vi "pump_motor_run.vi"(8 "error in (no error)":errorcluster, 9 "Enable":bool, 10 "Empty Swim Bladder":bool, 11 "PWM Duty Cycle [0, 1]":dbl(slide)=1.0 scale=0.0..1.0) -> (0 "error out":errorcluster, 1 "Driver Error/Pump Motor off":bool, 3 "Motor Current[A]":dbl)   [LabVIEW 2013]
uses:
  My Computer/Controls/Advanced Swimbladder Indicators.ctl
  <vilib>/myRIO/Instrument Drivers/Onboard IO/AI/vis/Smart Open.vi
  <vilib>/myRIO/Instrument Drivers/Onboard IO/AI/vis/Read.vi
  <vilib>/myRIO/Instrument Drivers/Onboard IO/DIO/vis/Smart Open.vi
  <vilib>/myRIO/Instrument Drivers/Onboard IO/DIO/vis/Read.vi
  <vilib>/myRIO/Instrument Drivers/Onboard IO/PWM/vis/Smart Open.vi
  <vilib>/myRIO/Instrument Drivers/Onboard IO/PWM/vis/Set Duty Cycle and Frequency.vi
  <vilib>/myRIO/Instrument Drivers/Onboard IO/DIO/vis/Write.vi
  <vilib>/myRIO/Instrument Drivers/Onboard IO/AI/vis/Open.vi
  <vilib>/myRIO/Instrument Drivers/Onboard IO/DIO/vis/Open.vi
  <vilib>/myRIO/Instrument Drivers/Onboard IO/PWM/vis/Open.vi
  <vilib>/myRIO/Common/Instrument Driver Framework/myRIO v1.0/AI/vis/myRIO v1.1 Open AI.vi
  <vilib>/myRIO/Common/Instrument Driver Framework/myRIO v1.0/DIO/vis/myRIO v1.1 Open DIO.vi
  <vilib>/myRIO/Common/Instrument Driver Framework/myRIO v1.0/PWM/vis/myRIO v1.1 Open PWM.vi
  <vilib>/myRIO/Common/Instrument Driver Framework/Utilities/vis/Validate Channels.vi
  <vilib>/myRIO/Common/Instrument Driver Framework/myRIO v1.0/AI/vis/myRIO v1.0 Reserve AI.vi
  <vilib>/myRIO/Common/Instrument Driver Framework/myRIO v1.0/DIO/vis/myRIO v1.0 Reserve DIO.vi
  <vilib>/myRIO/Common/Instrument Driver Framework/myRIO v1.0/PWM/vis/myRIO v1.0 Reserve PWM.vi
  <vilib>/myRIO/Common/Instrument Driver Framework/myRIO v1.0/AI/vis/myRIO v1.0 Build MUX Configuration AI.vi
  <vilib>/myRIO/Common/Instrument Driver Framework/myRIO v1.0/Resource Manager/vis/myRIO v1.0 Reserve Channel List.vi
  <vilib>/myRIO/Common/Instrument Driver Framework/myRIO v1.0/DIO/vis/myRIO v1.0 Build MUX Configuration DIO.vi
  <vilib>/myRIO/Common/Instrument Driver Framework/myRIO v1.0/PWM/vis/myRIO v1.0 Build MUX Configuration PWM.vi
  <vilib>/myRIO/Common/Instrument Driver Framework/myRIO v1.0/Resource Manager/vis/myRIO v1.0 Reserve Channel.vi
  <vilib>/myRIO/Common/Instrument Driver Framework/myRIO v1.0/Resource Manager/vis/myRIO v1.0 Unreserve Channel.vi
  <vilib>/myRIO/Common/Instrument Driver Framework/myRIO v1.0/Resource Manager/vis/myRIO v1.0 Create Configuration List.vi
  <vilib>/myRIO/Common/Instrument Driver Framework/myRIO v1.0/Resource Manager/vis/myRIO v1.0 Build Mutex Name.vi
  <vilib>/myRIO/Common/Instrument Driver Framework/myRIO v1.0/myRIO v1.1 Open.vi
  <vilib>/myRIO/Common/Instrument Driver Framework/myRIO v1.0/AI/vis/myRIO v1.0 Get Scaling Constants AI.vi
  <vilib>/Utility/VariantDataType/GetNumericInfo.vi
  <vilib>/Utility/error.llb/Error Cluster From Error Code.vi
  <vilib>/myRIO/Common/Instrument Driver Framework/Utilities/vis/IO Manager.vi
  <vilib>/myRIO/Common/Instrument Driver Framework/Utilities/vis/Configuration Manager.vi
  <vilib>/myRIO/Common/Instrument Driver Framework/myRIO v1.0/myRIO v1.0 Close.vi
  <vilib>/myRIO/Common/Instrument Driver Framework/myRIO v1.0/AI/vis/myRIO v1.0 Read AI.vi
  <vilib>/myRIO/Common/Instrument Driver Framework/myRIO v1.0/Resource Manager/vis/myRIO v1.0 Configure IO.vi
  <vilib>/myRIO/Common/Instrument Driver Framework/myRIO v1.0/DIO/vis/myRIO v1.0 Read DIO.vi
  <vilib>/myRIO/Common/Instrument Driver Framework/myRIO v1.0/PWM/vis/myRIO v1.0 Write PWM.vi
  <vilib>/myRIO/Common/Instrument Driver Framework/myRIO v1.0/DIO/vis/myRIO v1.0 Write DIO.vi
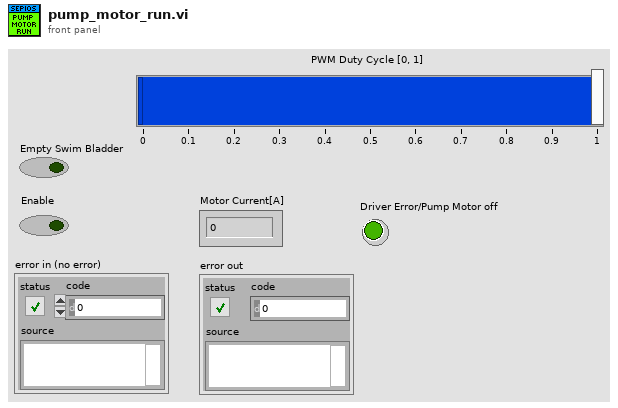
[diagram p1: front panel]
types:
  T1 = typedef "Advanced Swimbladder Indicators.ctl" = cluster{"P_ref [Pa]":dbl, "X_Actual [m]":dbl, "Motor Current[A]":dbl}
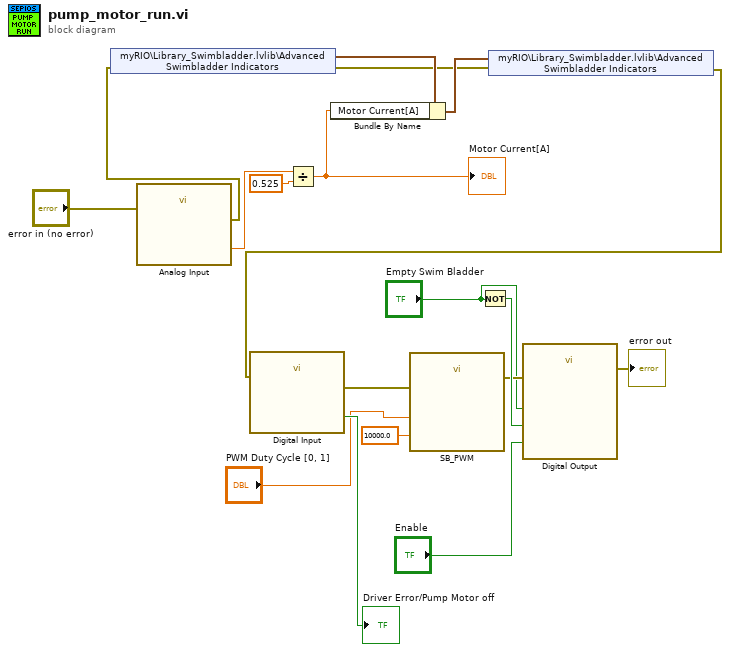
[diagram p0: block diagram]
diagram:
  n1 = call "Analog Input"("error in (no error)"="error in (no error)") -> ("SB_FB (B/AI0 (Pin 3))"=w14:dbl, "error out"=w3:errorcluster)  [unwired: 25 in]
  n2 = shared-variable "myRIO\\Library_Swimbladder.lvlib\\Advanced Swimbladder Indicators"(error in=w3) -> (w6:T1, error out=w2:errorcluster)
  n3 = Divide(x=w14, y=0.525) -> (x/y=w5:dbl)
  "Motor Current[A]" <- w5
  n4 = Bundle By Name(cluster=w6, "Motor Current[A]"=w5) -> (w4:T1)
  n5 = Not(x="Empty Swim Bladder") -> (.not. x?=w18:bool)
  n6 = shared-variable "myRIO\\Library_Swimbladder.lvlib\\Advanced Swimbladder Indicators"(w4, error in=w2) -> (error out=w1:errorcluster)
  n7 = call "Digital Input"("error in (no error)"=w1) -> ("SB_/SF (A/DIO13 (Pin 26))"=→"Driver Error/Pump Motor off":bool, "error out"=w12:errorcluster)  [unwired: 25 in]
  n8 = call "SB_PWM"("Duty Cycle (0-1)"="PWM Duty Cycle [0, 1]", "Frequency (Hz)"=10000.0, "error in (no error)"=w12) -> ("error out"=w11:errorcluster)  [unwired: 24 in]
  n9 = call "Digital Output"("SB_IN1 (A/DIO1 (Pin 13))"="Empty Swim Bladder", "SB_IN2 (A/DIO2 (Pin 15))"=w18, "SB_EN (A/DIO0 (Pin 11))"="Enable", "error in (no error)"=w11) -> ("error out"=→"error out":errorcluster)  [unwired: 23 in]
